vi "Unflatten From String.vi"(7 "iMessage in":refnum<class "iMessage.lvclass">, 8 "error in (no error)":errorcluster, 11 "binary string":string) -> (0 "error out":errorcluster, 3 "iMessage out":refnum<class "iMessage.lvclass">)   [LabVIEW 2017, in "Message Interface.lvlib" / "iMessage.lvclass"]
uses:
  iMessage.lvclass
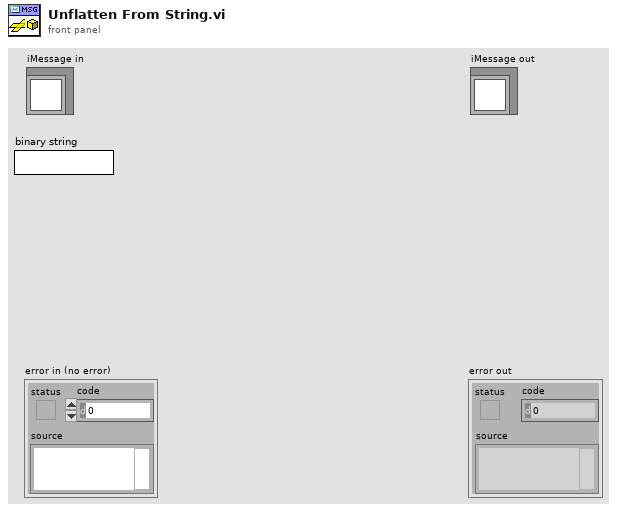
[diagram p1: front panel]
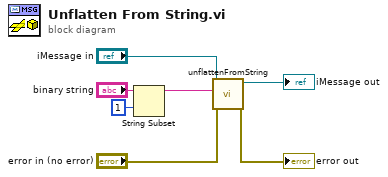
[diagram p0: block diagram]
diagram:
  n1 = String Subset(string="binary string", offset (0)=1) -> (substring=w2:string)  [unwired: 1 in]
  n2 = call-dynamic "unflattenFromString.vi"("error in (no error)"="error in (no error)", "binary string"=w2, "iMessage in"="iMessage in") -> ("error out"=→"error out":errorcluster, "iMessage out"=→"iMessage out":refnum<class "iMessage.lvclass">)  [unwired: 7 in]
